vi "PPMS magnet status.vi"(0 "GPIB address":string="15", 1 "Transmit Mode (0)":T1(ring), 2 "error in (no error)":errorcluster) -> (3 "Magnet Stable?":bool, 4 "Magnet Status":string, 5 "Status bits 4-7":i32, 6 "error out":errorcluster)   [LabVIEW 2018]
doc: "This checks the status of the PPMS magnet. If the magnet reports a stable field and the field is within .5% of the set field, Magnet stable? is set to TRUE, otherwise it is FALSE. It also returns a string containing the specific status of the magnet. bits 4-7 is the decimal value of the magnet status bits returned by the PPMS. See page A-7 for the meanings of various values."
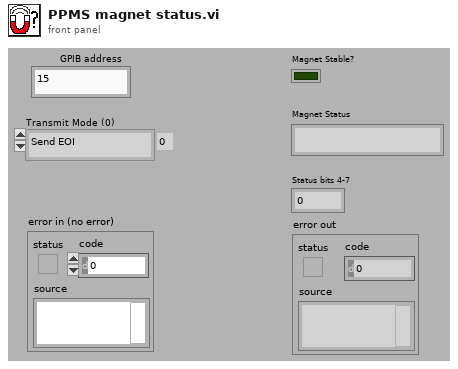
[diagram p1: front panel]
types:
  T1 = enum16{"Send EOI", "append CR w/ EOI", "append LF w/ EOI", "append CR LF w/ EOI", "append CR w/o EOI", "append LF w/o EOI", "append CR LF w/o EOI", "do not send EOI"}
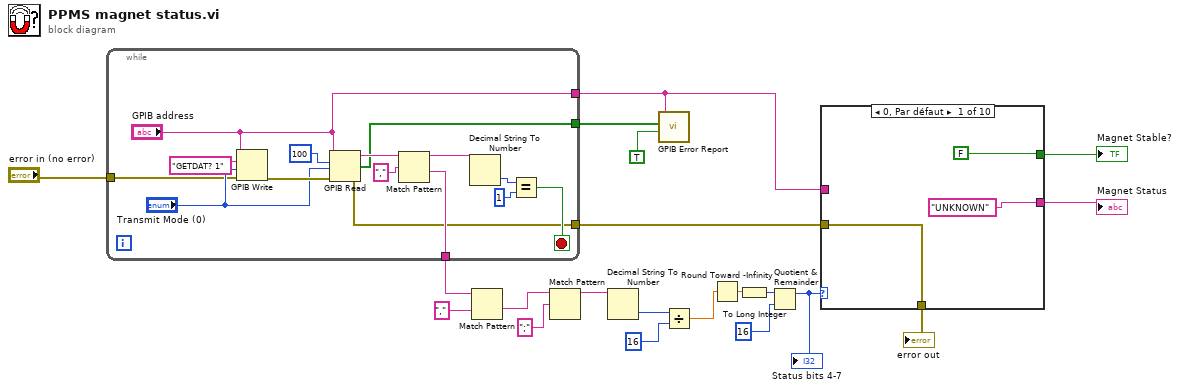
[diagram p0: block diagram]
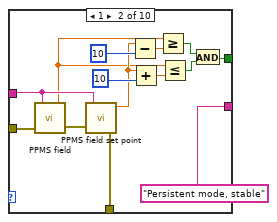
[diagram p2: hidden frame]
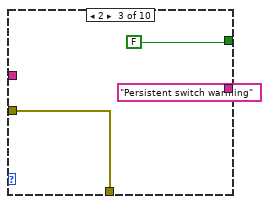
[diagram p3: hidden frame]
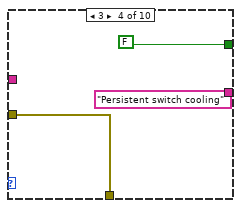
[diagram p4: hidden frame]
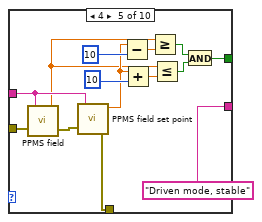
[diagram p5: hidden frame]
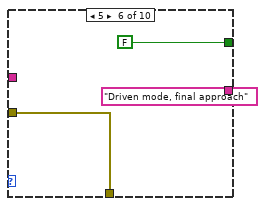
[diagram p6: hidden frame]
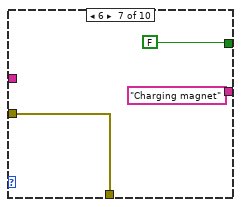
[diagram p7: hidden frame]
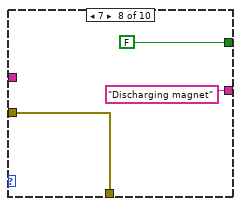
[diagram p8: hidden frame]
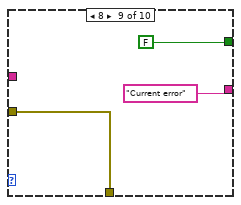
[diagram p9: hidden frame]
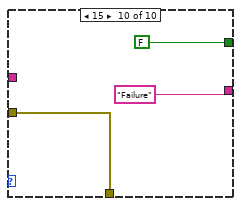
[diagram p10: hidden frame]
diagram:
  n1 = while {
    tunnel: [w25] -> w20
    tunnel: ["GPIB address"] -> w4
    tunnel: [w24] -> w14
    tunnel: "error in (no error)" -> [w22]
    tunnel: [w21] -> w2
    stop <- w26 stop-if-true
    n2 = GPIB Write(0:"GPIB address", 1:"GETDAT? 1", 2:"Transmit Mode (0)", 3:w22) -> (6:w34:errorcluster)  [unwired: 1 in, 1 out]
    n3 = GPIB Read(0:"GPIB address", 1:100, 2:"Transmit Mode (0)", 3:w34) -> (5:w31:string, 6:w24:bool[], 7:w21:errorcluster)  [unwired: 1 in]
    n4 = Match Pattern(string=w31, regular expression=",") -> (before substring=w29:string, after substring=w25:string)  [unwired: 1 in, 2 out]
    n5 = Decimal String To Number(string=w29) -> (number=w28:i32)  [unwired: 2 in, 1 out]
    n6 = Equal?(x=w28, y=1) -> (x = y?=w26:bool)
  }
  n7 = Match Pattern(string=w20, regular expression=",") -> (after substring=w18:string)  [unwired: 1 in, 3 out]
  n8 = Match Pattern(string=w18, regular expression=";") -> (before substring=w16:string)  [unwired: 1 in, 3 out]
  n9 = Decimal String To Number(string=w16) -> (number=w9:i32)  [unwired: 2 in, 1 out]
  n10 = call "GPIB Error Report.vi"("Dialog?(F)"=TRUE, "Status"=w14, "Address String"=w4) -> ()  [unwired: 1 in, 2 out]
  n11 = Divide(x=w9, y=16) -> (x/y=w8:dbl)
  n12 = Round Toward -Infinity(1:w8) -> (0:w7:dbl)
  n13 = To Long Integer(number=w7) -> (32bit integer=w6:i32)
  n14 = Quotient & Remainder(x=w6, y=16) -> (x-y*floor(x/y)=w11:i32)  [unwired: 1 out]
  "Status bits 4-7" <- w11
  n15 = case shown="0, Par défaut" w11 {
    tunnel: ["UNKNOWN" "Persistent mode, stable" "Persistent switch warming" "Persistent switch cooling" "Driven mode, stable" "Driven mode, final approach" "Charging magnet" "Discharging magnet" "Current error" "Failure"] -> w15
    tunnel: [FALSE w43 FALSE FALSE w70 FALSE FALSE FALSE FALSE FALSE] -> w12
    tunnel: w4 -> [_ w42 _ _ w65 _ _ _ _ _]
    tunnel: w2 -> [w36 w40 w53 w56 w60 w73 w76 w79 w82 w85]
    tunnel: [w36 w39 w53 w56 w59 w73 w76 w79 w82 w85] -> w1
    frame 0, Default {
    }
    frame 1 {
      n16 = call "PPMS field.vi"("error in (no error)"=w40, "GPIB address"=w42) -> ("error out"=w51:errorcluster, "Field (Oe)"=w41:dbl)  [unwired: 1 in]
      n17 = call "PPMS field set point.vi"("GPIB address"=w42, "error in (no error)"=w51) -> ("Field set point (Oe)"=w44:dbl, "error out"=w39:errorcluster)  [unwired: 2 out]
      n18 = Subtract(x=w44, y=10) -> (x-y=w48:dbl)
      n19 = Add(x=w44, y=10) -> (x+y=w47:dbl)
      n20 = Greater Or Equal?(x=w41, y=w48) -> (x >= y?=w50:bool)
      n21 = Less Or Equal?(x=w41, y=w47) -> (x <= y?=w49:bool)
      n22 = And(x=w50, y=w49) -> (x .and. y?=w43:bool)
    }
    frame 2 {
    }
    frame 3 {
    }
    frame 4 {
      n23 = call "PPMS field.vi"("error in (no error)"=w60, "GPIB address"=w65) -> ("error out"=w71:errorcluster, "Field (Oe)"=w61:dbl)  [unwired: 1 in]
      n24 = call "PPMS field set point.vi"("GPIB address"=w65, "error in (no error)"=w71) -> ("Field set point (Oe)"=w62:dbl, "error out"=w59:errorcluster)  [unwired: 2 out]
      n25 = Subtract(x=w62, y=10) -> (x-y=w67:dbl)
      n26 = Add(x=w62, y=10) -> (x+y=w66:dbl)
      n27 = Greater Or Equal?(x=w61, y=w67) -> (x >= y?=w69:bool)
      n28 = Less Or Equal?(x=w61, y=w66) -> (x <= y?=w68:bool)
      n29 = And(x=w69, y=w68) -> (x .and. y?=w70:bool)
    }
    frame 5 {
    }
    frame 6 {
    }
    frame 7 {
    }
    frame 8 {
    }
    frame 15 {
    }
  }
  "Magnet Status" <- w15
  "Magnet Stable?" <- w12
  "error out" <- w1
